vi "Degrees To Ticks.vi"(11 "Steering Angles (degrees)":T1) -> (3 "Steering Angles (ticks)":T1)   [LabVIEW 2020]
doc: "unit conversion: degrees --> ticks (multiplying)"
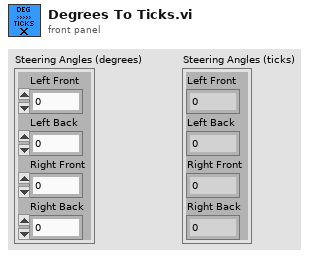
[diagram p1: front panel]
types:
  T1 = cluster{"Left Front":dbl, "Left Back":dbl, "Right Front":dbl, "Right Back":dbl}
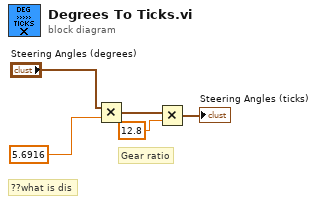
[diagram p0: block diagram]
diagram:
  # "??what is dis"
  # "Gear ratio"
  n1 = Multiply(x="Steering Angles (degrees)", y=5.6916 ("scale factor")) -> (x*y=w5:T1)
  n2 = Multiply(x=w5, y=12.8) -> (x*y=→"Steering Angles (ticks)":T1)
